vi "createNewLog.vi"(8 "error in (no error)":errorcluster, 11 "Model in":refnum<class "Model.lvclass">) -> (0 "error out":errorcluster, 3 "Model out":refnum<class "Model.lvclass">)   [LabVIEW 2013, in "Model.lvclass"]
uses:
  Model.lvclass
  Model.lvclass/Model.ctl
  ApplicationElements/Log/TestDataLog/TestDataLog.lvclass
  UserEvents/UserEvents.lvclass/UserEvents.ctl
  <userlib>/Common/Log/Log/Log.lvclass/Log.ctl
  <userlib>/Common/Log/Log/Log.lvclass
  UserEvents/UserEvents.lvclass
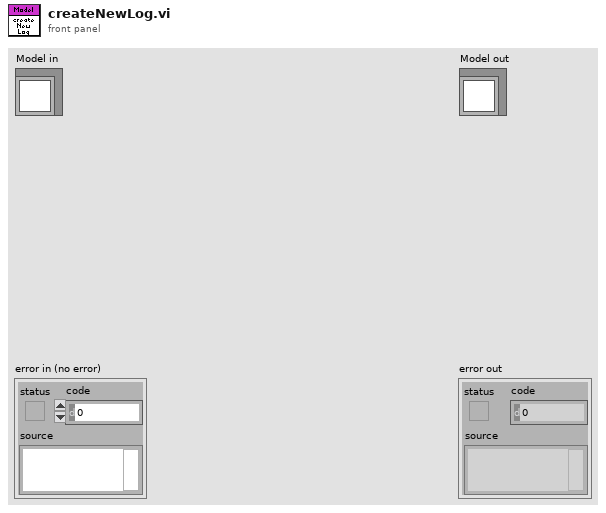
[diagram p1: front panel]
types:
  T1 = typedef "M2AADTTypedefs.lvlib/PubDataEvents.ctl" = cluster{"State":refnum<user-event>, "ErrorCode":refnum<user-event>, "OutputData":refnum<user-event>, "InputData":refnum<user-event>, "TestStatus":refnum<user-event>, "LogPath":refnum<user-event>}
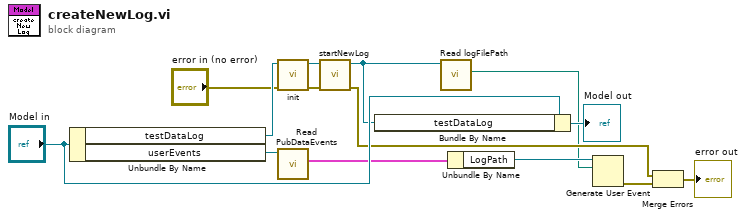
[diagram p0: block diagram]
diagram:
  n1 = Unbundle By Name("Model in") -> ("testDataLog"=w4:refnum<class "TestDataLog.lvclass">, "userEvents"=w7:refnum<class "UserEvents.lvclass">)
  n2 = call-dynamic "init.vi"("error in (no error)"="error in (no error)", "Logger in"=w4) -> ("error out"=w2:errorcluster, "Logger out"=w3:refnum<class "TestDataLog.lvclass">)  [unwired: 8 in]
  n3 = call "Read PubDataEvents.vi"("UserEvents in"=w7) -> ("PubDataEvents"=w9:T1)  [unwired: 9 in, 1 out]
  n4 = call <userlib>:"startNewLog.vi"("error in (no error)"=w2, "Logger in"=w3) -> ("error out"=w12:errorcluster, "Logger out"=w5:refnum<class "TestDataLog.lvclass">)  [unwired: 8 in]
  n5 = Bundle By Name(cluster="Model in", "testDataLog"=w5) -> (→"Model out":refnum<class "Model.lvclass">)
  n6 = call <userlib>:"Read logFilePath.vi"("Logger in"=w5) -> ("logFilePath"=w6:path)  [unwired: 9 in, 1 out]
  n7 = Unbundle By Name(w9) -> ("LogPath"=w8:refnum<user-event>)
  n8 = Generate User Event(user event=w8, event data cluster=w6) -> (error out=w11:errorcluster)  [unwired: 2 in, 1 out]
  n9 = Merge Errors(w12, w11) -> (→"error out":errorcluster)
